vi "EOL Check Initial Motion.vi"(6 "Motor Type":T1, 7 "Station Index":i32, 8 "Error Table In":string[][](array[string]), 9 "Current Motion":T2, 10 "Current Data Index":i32, 11 "Current Data":sgl[][](array[numeric])) -> (0 "Error Table":string[][](array[string]), 1 "Pass?":bool, 2 "Current Data Index Out":i32, 3 "Current Data Out":sgl[][](array[numeric]))   [LabVIEW 2018]
uses:
  02.Type Def's/All Motions.ctl
  05.UserVI's/type defs/EOL Motor Type.ctl
  <vilib>/measure/mamon.llb/Trigger Detection for 1 Channel.vi
  <vilib>/measure/NI_MAPro.lvlib
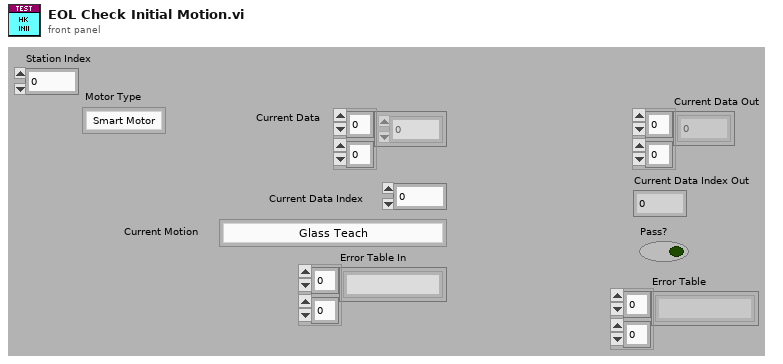
[diagram p1: front panel]
types:
  T1 = typedef "EOL Motor Type.ctl" = enum16{"Smart Motor", "Sensor Motor"}
  T2 = typedef "All Motions.ctl" = enum16{"Glass Teach", "Glass Slide Open", "Glass Slide Close", "Glass Vent Open", "Glass Vent Close", "Sunshade Teach", "Sunshade Open", "Sunshade Close", "Idle", "Sunshade Open 2", "Sunshade Close 2", "Glass Slide Open Sunshade Open", "Glass Slide Open Sunshade Close", "Glass Slide Close Sunshade Open", "Glass Slide Close Sunshade Close", "Glass Vent Open Sunshade Open", "Glass Vent Open Sunshade Close", "Glass Vent Close Sunshade Open", "Glass Vent Close Sunshade Close", "Express Glass Slide Open", "Express Glass Slide Close", "Express Glass Vent Open", "Express Glass Vent Close", "Express Sunshade Open", "Express Sunshade Close", "Express Sunshade Open 2", "Express Sunshade Close 2", "Express Glass Slide Open Sunshade Open", "Express Glass Slide Open Sunshade Close", "Express Glass Slide Close Sunshade Open", "Express Glass Slide Close Sunshade Close", "Express Glass Vent Open Sunshade Open", "Express Glass Vent Open Sunshade Close", "Express Glass Vent Close Sunshade Open", "Express Glass Vent Close Sunshade Close", "Goto Position Glass", "Goto Position Sunshade", "Sunshade Teach 2"}
  T3 = typedef "EOL Analog Input Control.ctl" = enum16{"SW PS  Volage", "Switch A", "Switch B", "Switch C", "Motor Voltage", "Motor Current", "ATS"}
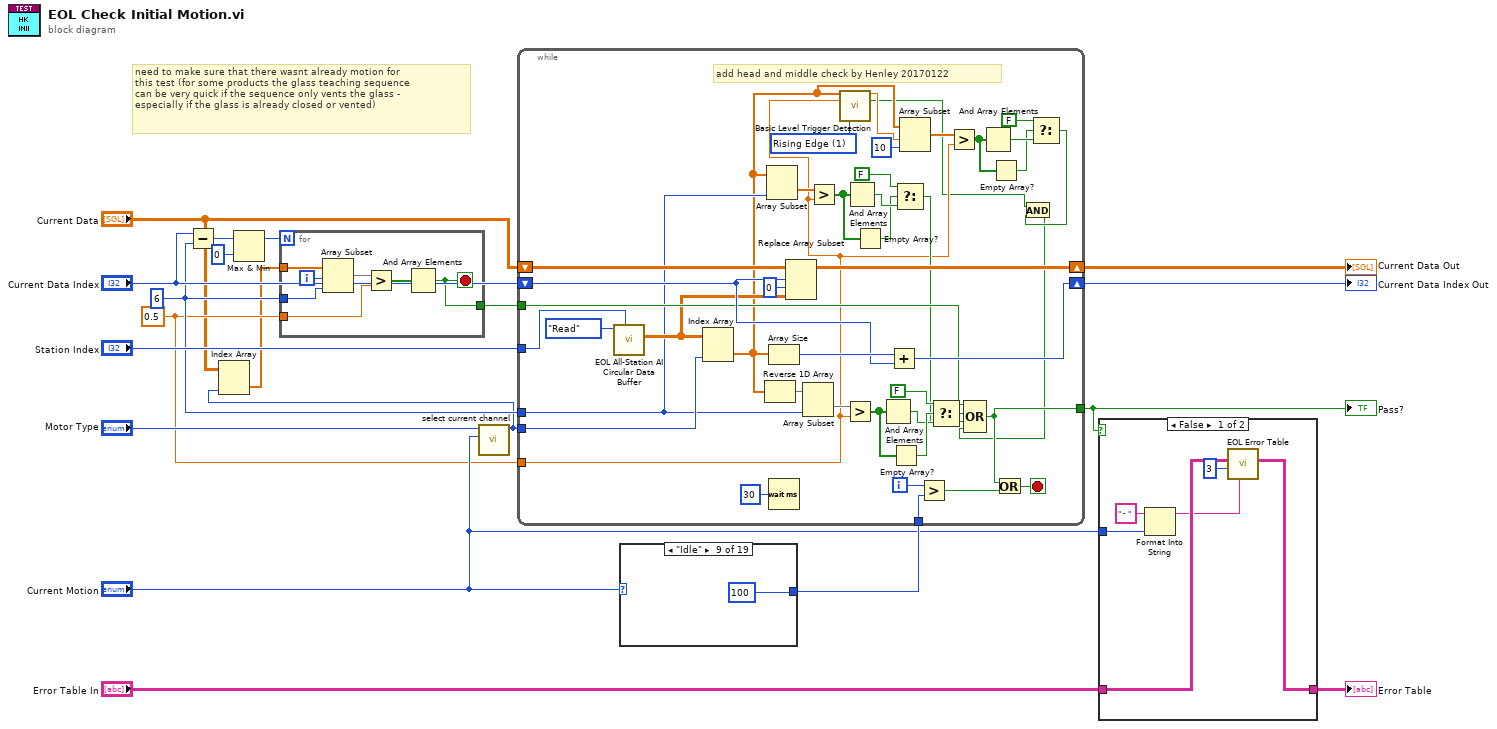
[diagram p0: block diagram]
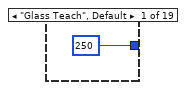
[diagram p2: hidden frame]
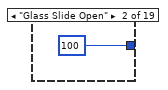
[diagram p3: hidden frame]
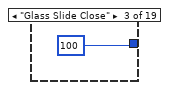
[diagram p4: hidden frame]
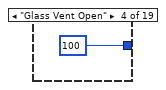
[diagram p5: hidden frame]
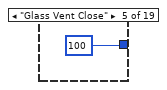
[diagram p6: hidden frame]
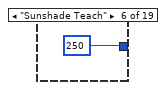
[diagram p7: hidden frame]
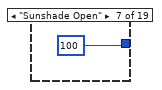
[diagram p8: hidden frame]
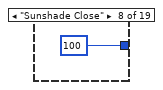
[diagram p9: hidden frame]
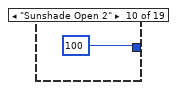
[diagram p10: hidden frame]
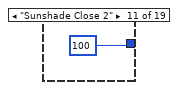
[diagram p11: hidden frame]
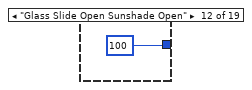
[diagram p12: hidden frame]
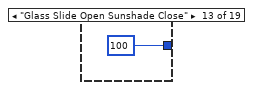
[diagram p13: hidden frame]
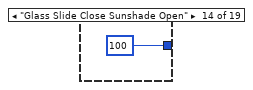
[diagram p14: hidden frame]
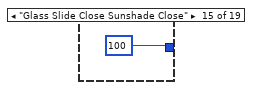
[diagram p15: hidden frame]
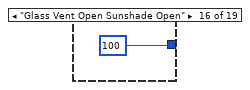
[diagram p16: hidden frame]
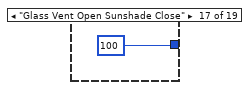
[diagram p17: hidden frame]
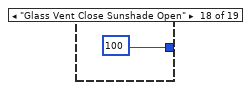
[diagram p18: hidden frame]
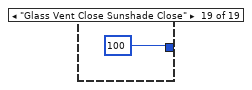
[diagram p19: hidden frame]
diagram:
  w5 = sgl 0.5 ("y")
  w9 = 6 ("length")
  # "need to make sure that there wasnt already motion for\nthis test (for some products the glass teaching sequence \ncan be very quick if the sequence only vents the glass - \nespecially if the glass is already closed or vented)"
  n1 = Subtract(x="Current Data Index", y=w9) -> (x-y=w8:i32)
  n2 = Max & Min(x=w8, y=0) -> (max(x,y)=w6:i32)  [unwired: 1 out]
  n3 = call "select current channel.vi"("Current Motion"="Current Motion", "Motor Type"="Motor Type") -> ("Analog channel"=w1:T3)  [unwired: 9 in]
  n4 = Index Array(array="Current Data", index (col)=w1) -> (element=w2:sgl[])  [unwired: 1 in]
  n5 = for {
    N: w6 -> [_]
    tunnel: w2 -> [w26]
    tunnel: w9 -> [w24]
    tunnel: w5 -> [w21]
    tunnel: [w20] -> w4
    i -> [w25]
    stop <- w20 stop-if-true
    n6 = Array Subset(array=w26, index=w25, length=w24) -> (w22:sgl[])
    n7 = Greater?(x=w22, y=w21) -> (0:w23:bool[])
    n8 = And Array Elements(Boolean array=w23) -> (logical AND=w20:bool)
  }
  n9 = case shown="\"Idle\"" "Current Motion" {
    tunnel: [250 ("y") 100 ("y") 100 ("y") 100 ("y") 100 ("y") 250 ("y") 100 ("y") 100 ("y") 100 ("y") 100 ("y") 100 ("y") 100 ("y") 100 ("y") 100 ("y") 100 ("y") 100 ("y") 100 ("y") 100 ("y") 100 ("y")] -> w14
    frame "Glass Teach", Default {
    }
    frame "Glass Slide Open" {
    }
    frame "Glass Slide Close" {
    }
    frame "Glass Vent Open" {
    }
    frame "Glass Vent Close" {
    }
    frame "Sunshade Teach" {
    }
    frame "Sunshade Open" {
    }
    frame "Sunshade Close" {
    }
    frame "Idle" {
    }
    frame "Sunshade Open 2" {
    }
    frame "Sunshade Close 2" {
    }
    frame "Glass Slide Open Sunshade Open" {
    }
    frame "Glass Slide Open Sunshade Close" {
    }
    frame "Glass Slide Close Sunshade Open" {
    }
    frame "Glass Slide Close Sunshade Close" {
    }
    frame "Glass Vent Open Sunshade Open" {
    }
    frame "Glass Vent Open Sunshade Close" {
    }
    frame "Glass Vent Close Sunshade Open" {
    }
    frame "Glass Vent Close Sunshade Close" {
    }
  }
  n10 = while {
    tunnel: [w72] -> w15
    shift-right: [w81] -> w19
    shift-left: "Current Data Index" -> [w83]
    shift-right: [w77] -> w18
    shift-left: "Current Data" -> [w82]
    tunnel: "Station Index" -> [w75]
    tunnel: w14 -> [w76]
    tunnel: w1 -> [w73]
    tunnel: w9 -> [w60]
    tunnel: w4 -> [w71]
    tunnel: w5 -> [w53]
    i -> [w87]
    stop <- w85 stop-if-true
    w58 = u16 1 items=["Falling Edge", "Rising Edge"] ("trigger slope")
    # "add head and middle check by Henley 20170122"
    n11 = call "EOL All-Station AI Circular Data Buffer.vi"("station idx"=w75, "Mode"=enum16{"Initialize", "Read", "Write"}."Read") -> ("Data Read (Samp-Ro, Ch-Col)"=w67:sgl[][])  [unwired: 9 in]
    n12 = Index Array(array=w67, index (col)=w73) -> (element=w57:sgl[])  [unwired: 1 in]
    n13 = Reverse 1D Array(array=w57) -> (reversed array=w89:sgl[])
    n14 = Array Subset(array=w57, length=w60) -> (w63:sgl[])  [unwired: 1 in]
    n15 = Array Size(array=w57) -> (size(s)=w84:i32)
    n16 = Wait (ms)(milliseconds to wait=u32 30) -> ()  [unwired: 1 out]
    n17 = Replace Array Subset(array=w82, new element=w67, index (row)=w83, index (col)=0 ("disabled index (col)")) -> (w77:sgl[][])
    n18 = Array Subset(array=w89, length=w60) -> (w70:sgl[])  [unwired: 1 in]
    n19 = Greater?(x=w63, y=w53) -> (0:w64:bool[])
    n20 = call-poly <vilib>:"Basic Level Trigger Detection.vi"("signal in"=w57, "level"=w53, "trigger slope"=w58) -> ("trigger location"=w55:dbl, "trigger detected?"=w48:bool)  [unwired: 10 in, 1 out]
    n21 = Greater?(x=w70, y=w53) -> (0:w69:bool[])
    n22 = And Array Elements(Boolean array=w64) -> (logical AND=w65:bool)
    n23 = Empty Array?(array=w64) -> (empty?=w61:bool)
    n24 = And Array Elements(Boolean array=w69) -> (logical AND=w68:bool)
    n25 = Add(x=w84, y=w83) -> (x+y=w81:i32)
    n26 = Empty Array?(array=w69) -> (empty?=w79:bool)
    n27 = Select(t=FALSE, s=w61, f=w65) -> (s? t:f=w59:bool)
    n28 = Array Subset(array=w57, index=w55, length=10) -> (w54:sgl[])
    n29 = Greater?(x=w87, y=w76) -> (0:w86:bool)
    n30 = Select(t=FALSE, s=w79, f=w68) -> (s? t:f=w80:bool)
    n31 = Greater?(x=w54, y=w53) -> (0:w49:bool[])
    n32 = And Array Elements(Boolean array=w49) -> (logical AND=w52:bool)
    n33 = Empty Array?(array=w49) -> (empty?=w50:bool)
    n34 = Select(t=FALSE, s=w50, f=w52) -> (s? t:f=w47:bool)
    n35 = And(x=w48, y=w47) -> (x .and. y?=w46:bool)
    n36 = Compound Arithmetic op=OR(w71, w80, w59, w46) -> (w72:bool)
    n37 = Or(x=w72, y=w86) -> (x .or. y?=w85:bool)
  }
  "Current Data Index Out" <- w19
  "Current Data Out" <- w18
  "Pass?" <- w15
  n38 = case shown="False" w15 {
    tunnel: "Error Table In" -> [w95 w96]
    tunnel: [w90 w96] -> w17
    tunnel: "Current Motion" -> [w94 _]
    frame False {
      n39 = Format Into String(initial string=" - ", w94) -> (resulting string=w92:string)  [unwired: 2 in, 1 out]
      n40 = call "EOL Error Table.vi"("Error Description"=w92, "Error No."=u16 3, "Error Table In"=w95) -> ("Error Table Out"=w90:string[][])  [unwired: 7 in, 1 out]
    }
    frame True {
    }
  }
  "Error Table" <- w17
